vi "CleanupFlexUIActorMakerReferences.vi"(8 "error in (no error)":errorcluster, 11 "FlexUIActorMaker in":refnum<class "FlexUIActorMaker.lvclass">) -> (0 "error out":errorcluster, 3 "FlexUIActorMaker out":refnum<class "FlexUIActorMaker.lvclass">)   [LabVIEW 2016, in "FlexUIActorMaker.lvlib" / "FlexUIActorMaker.lvclass"]
uses:
  FlexUIActorMaker.lvclass
  FlexUIActorMaker.lvclass/FlexUIActorMaker.ctl
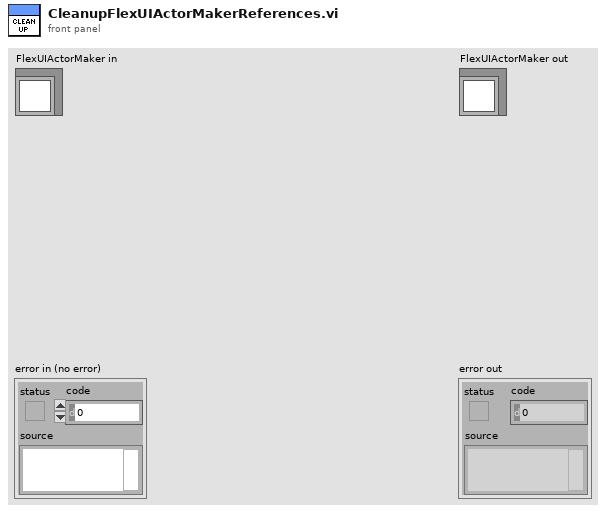
[diagram p1: front panel]
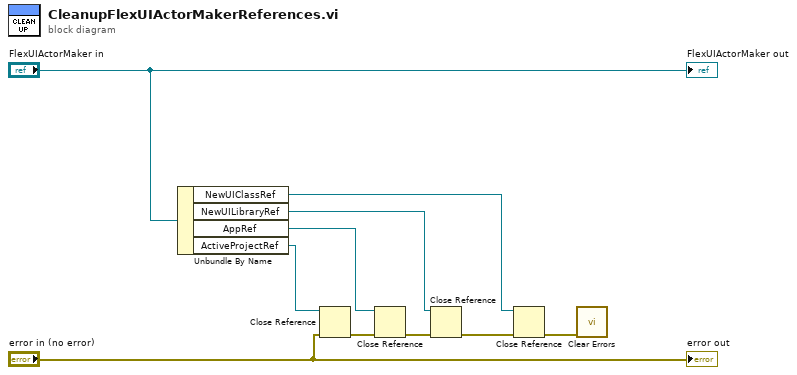
[diagram p0: block diagram]
diagram:
  n1 = Unbundle By Name("FlexUIActorMaker in") -> ("NewUIClassRef"=w3:refnum<vi>, "NewUILibraryRef"=w4:refnum<vi>, "AppRef"=w5:refnum<vi>, "ActiveProjectRef"=w8:refnum<vi>)
  n2 = Close Reference(reference=w8, error in (no error)="error in (no error)") -> (error out=w9:errorcluster)
  n3 = Close Reference(reference=w5, error in (no error)=w9) -> (error out=w6:errorcluster)
  n4 = Close Reference(reference=w4, error in (no error)=w6) -> (error out=w7:errorcluster)
  n5 = Close Reference(reference=w3, error in (no error)=w7) -> (error out=w2:errorcluster)
  n6 = call <vilib>:"Clear Errors.vi"("error in (no error)"=w2) -> ()  [unwired: 5 in, 2 out]
  "error out" <- "error in (no error)"
  "FlexUIActorMaker out" <- "FlexUIActorMaker in"
